vi "GetImage 1.vi"(0 "XRef":T4, 1 "State In":T3) -> (14 "Image":T2, 15 "Fatal Error Out":T1)   [LabVIEW 2013, in "VireoFunctionNode.xnode"]
uses:
  VireoFunctionNode.xnode
  <vilib>/XNodeSupport/XNodeXNodeRef.ctl
  State 1.ctl
  <vilib>/XNodeSupport/XNodeImage.ctl
  <vilib>/XNodeSupport/XNodeErrorCluster.ctl
  <vilib>/Utility/VariantDataType/VariantType.lvlib
  <vilib>/XNodeSupport/NI_XNodeSupport.lvlib
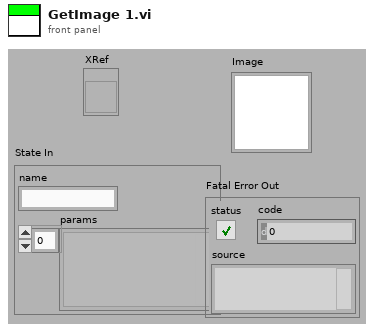
[diagram p1: front panel]
types:
  T1 = typedef "NI_XNodeSupport.lvlib/XNodeErrorCluster.ctl" = errorcluster
  T2 = typedef "NI_XNodeSupport.lvlib/XNodeImage.ctl" = picture
  T3 = typedef "VireoFunctionNode.xnode/State 1.ctl" = cluster{"name":string, "params":variant[]}
  T4 = typedef "NI_XNodeSupport.lvlib/XNodeXNodeRef.ctl" = refnum<vi>
  T5 = cluster{"left":i16, "top":i16, "right":i16, "bottom":i16}
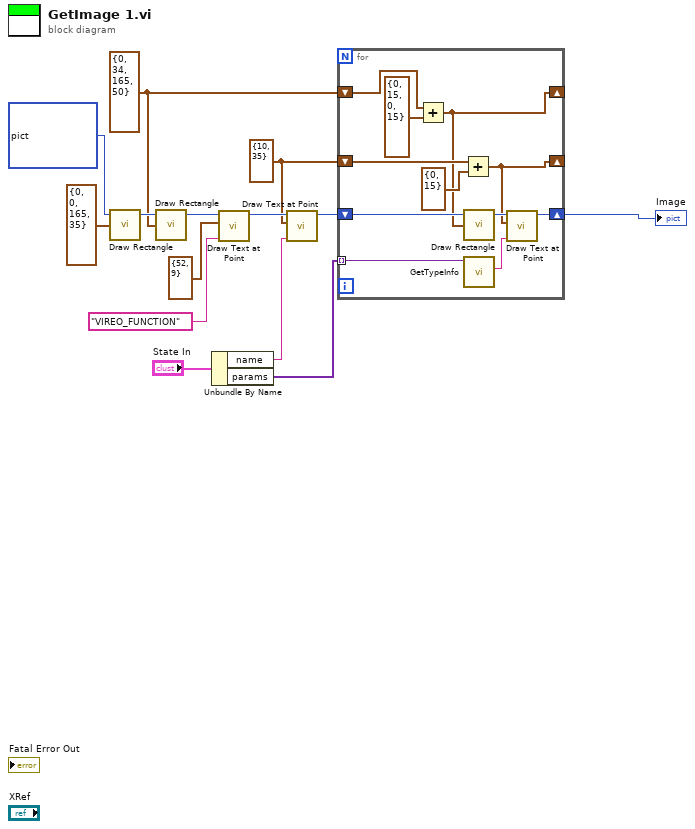
[diagram p0: block diagram]
diagram:
  w2 = T5 {"left"=0, "top"=34, "right"=165, "bottom"=50} ("rect")
  w3 = cluster{"x":i16, "y":i16} {"x"=10, "y"=35} ("origin")
  n1 = call <vilib>:"Draw Rectangle.vi"("picture"=picture bytes[5232] ("new picture"), "rect"=T5 {"left"=0, "top"=0, "right"=165, "bottom"=35}) -> ("new picture"=w7:picture)  [unwired: 7 in]
  n2 = call <vilib>:"Draw Rectangle.vi"("picture"=w7, "rect"=w2) -> ("new picture"=w6:picture)  [unwired: 7 in]
  n3 = Unbundle By Name("State In") -> ("name"=w8:string, "params"=w4:variant[])
  n4 = call <vilib>:"Draw Text at Point.vi"("text"="VIREO_FUNCTION", "origin"=cluster{"x":i16, "y":i16} {"x"=52, "y"=9}, "picture"=w6) -> ("new picture"=w10:picture)  [unwired: 7 in, 1 out]
  n5 = call <vilib>:"Draw Text at Point.vi"("text"=w8, "origin"=w3, "picture"=w10) -> ("new picture"=w5:picture)  [unwired: 7 in, 1 out]
  n6 = for {
    shift-right: [w21] -> w1
    shift-left: w5 -> [w20]
    tunnel: w4 -> [w25] mode=indexing
    shift-right: [w18] -> _
    shift-left: w3 -> [w23]
    shift-right: [w15] -> _
    shift-left: w2 -> [w17]
    n7 = Add(x=w17, y=T5 {"left"=0, "top"=15, "right"=0, "bottom"=15}) -> (x+y=w15:T5)
    n8 = Add(x=w23, y=cluster{"x":i16, "y":i16} {"x"=0, "y"=15}) -> (x+y=w18:cluster{"x":i16, "y":i16})
    n9 = call <vilib>:"Draw Rectangle.vi"("picture"=w20, "rect"=w15) -> ("new picture"=w19:picture)  [unwired: 7 in]
    n10 = call <vilib>:"GetTypeInfo.vi"("Variant"=w25) -> ("Name"=w22:string)  [unwired: 6 in, 4 out]
    n11 = call <vilib>:"Draw Text at Point.vi"("text"=w22, "origin"=w18, "picture"=w19) -> ("new picture"=w21:picture)  [unwired: 7 in, 1 out]
  }
  "Image" <- w1
